vi "BRig_dataExp_T_ENLPenalty.vi"() -> (2 "output_ENL_penalty":i32)   [LabVIEW 2014]
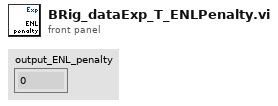
[diagram p1: front panel]
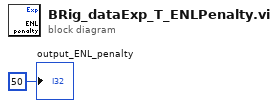
[diagram p0: block diagram]
diagram:
  "output_ENL_penalty" <- 50 ("output_iBlock")
